vi "CRYPART REMOVE FRAME.vi"(10 "tFrame":T2) -> (2 "tFrame_Out":T2)   [LabVIEW 2013]
uses:
  <vilib>/Utility/miscctls.llb/LVRectTypeDef.ctl
  CRYMain Sub Window Global.vi
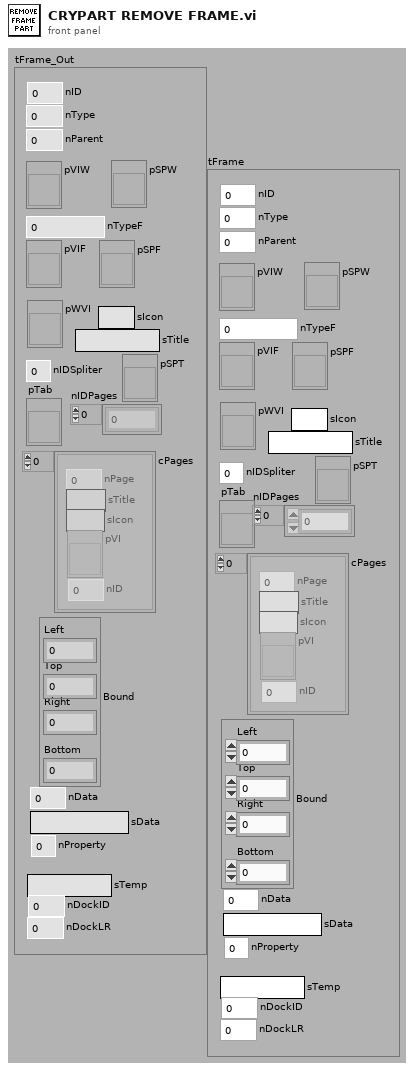
[diagram p1: front panel]
types:
  T1 = typedef "LVRectTypeDef.ctl" = cluster{"Left":i16, "Top":i16, "Right":i16, "Bottom":i16}
  T2 = cluster{"nType":i32, "nParent":i32, "pVIW":refnum<vi>, "pSPW":refnum<vi>, "nTypeF":i32, "pVIF":refnum<vi>, "pSPF":refnum<vi>, "nIDSpliter":i32, "nProperty":i32, "Bound":T1, "nID":i32, "nData":i32, "sData":string, "pWVI":refnum<vi>, "sTitle":string, "cPages":cluster{"nPage":i32, "sTitle":string, "sIcon":string, "pVI":refnum<vi>, "nID":i32}[], "pTab":refnum<vi>, "nIDPages":i32[], "pSPT":refnum<vi>, "sTemp":string, "nDockID":i32, "nDockLR":i32, "sIcon":string}
  T3 = cluster{"CLOSE_HIDE":i32, "CLOSE_CLOSE":i32, "DOCK_ENABLE":i32, "DOCK_DISABLE":i32, "FOCUS_SHOW":i32, "FOCUS_HIDE":i32}
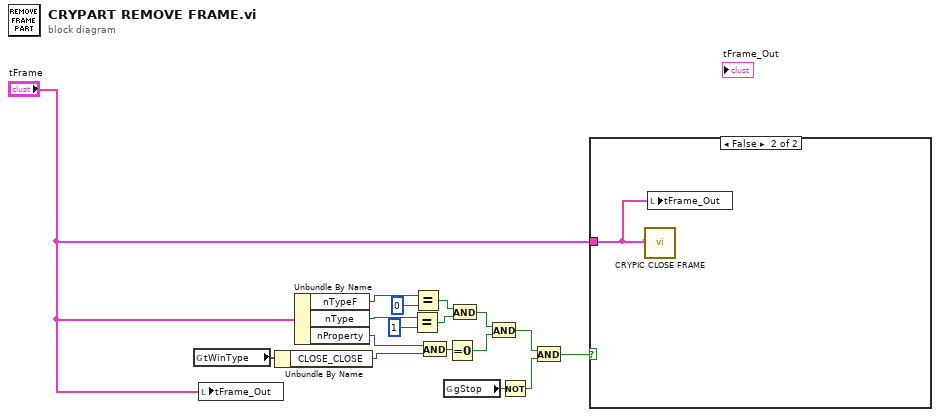
[diagram p0: block diagram]
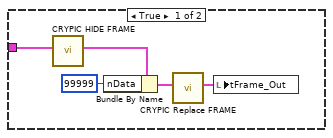
[diagram p2: hidden frame]
diagram:
  n1 = global read "CRYMain Sub Window Global.vi" "tWinType"() -> (w17:T3)
  n2 = local write "tFrame_Out"("tFrame") -> ()
  n3 = Unbundle By Name(w17) -> ("CLOSE_CLOSE"=w16:i32)
  n4 = Unbundle By Name("tFrame") -> ("nTypeF"=w11:i32, "nType"=w13:i32, "nProperty"=w15:i32)
  n5 = Equal?(x=w13, y=1) -> (x = y?=w9:bool)
  n6 = Equal?(x=w11, y=0) -> (x = y?=w8:bool)
  n7 = And(x=w15, y=w16) -> (x .and. y?=w14:i32)
  n8 = global read "CRYMain Sub Window Global.vi" "gStop"() -> (w4:bool)
  n9 = Equal To 0?(x=w14) -> (x = 0?=w6:bool)
  n10 = And(x=w8, y=w9) -> (x .and. y?=w7:bool)
  n11 = And(x=w7, y=w6) -> (x .and. y?=w5:bool)
  n12 = Not(x=w4) -> (.not. x?=w3:bool)
  n13 = And(x=w5, y=w3) -> (x .and. y?=w2:bool)
  n14 = case shown="False" w2 {
    tunnel: "tFrame" -> [w22 w23]
    frame True {
      n15 = call "CRYPIC HIDE FRAME.vi"("tFrame"=w22) -> ("tFrame_Out"=w21:T2)  [unwired: 10 in]
      n16 = Bundle By Name(cluster=w21, "nData"=99999) -> (w19:T2)
      n17 = call "CRYPIC Replace FRAME.vi"("tFrame"=w19) -> ("tFrame_Out"=w18:T2)  [unwired: 10 in]
      n18 = local write "tFrame_Out"(w18) -> ()
    }
    frame False {
      n19 = call "CRYPIC CLOSE FRAME.vi"("tFrame"=w23) -> ()  [unwired: 11 in]
      n20 = local write "tFrame_Out"(w23) -> ()
    }
  }
